vi "database MS Access test.vi"() -> ()   [LabVIEW 2020]
uses:
  source/Database OOP/Database Interfaces/Column Information.ctl
  source/Database OOP/Database Interfaces/Database data type.ctl
  source/Database OOP/ADODB/ADODB Class/ADODB.lvclass
  source/Database OOP/ADODB/UDL Connection Class/UDL Connection.lvclass
  C:/Users/User/Desktop/Raman Program/Database OOP/source/Database OOP/Database Interfaces/Database Connection Class/Database Connection.lvclass
  source/Database OOP/Database Interfaces/Database Advanced Schema Class/Database Adv Schema.lvclass
  source/Database OOP/Database Interfaces.lvlib
panel:
  out "Provider Name":string
  out "Timestamp":string[](array[string])
  out "Column Information Array 2":T1[](array[typedef])
  out "Primary Key Array":string[](array[string])
  out "Column Information Array":T1[](array[typedef])
  out "Foreign Key Array":T3(array[cluster])
  out "Column Name Array":string[](array[string])
  out "Table Names":string[](array[string])
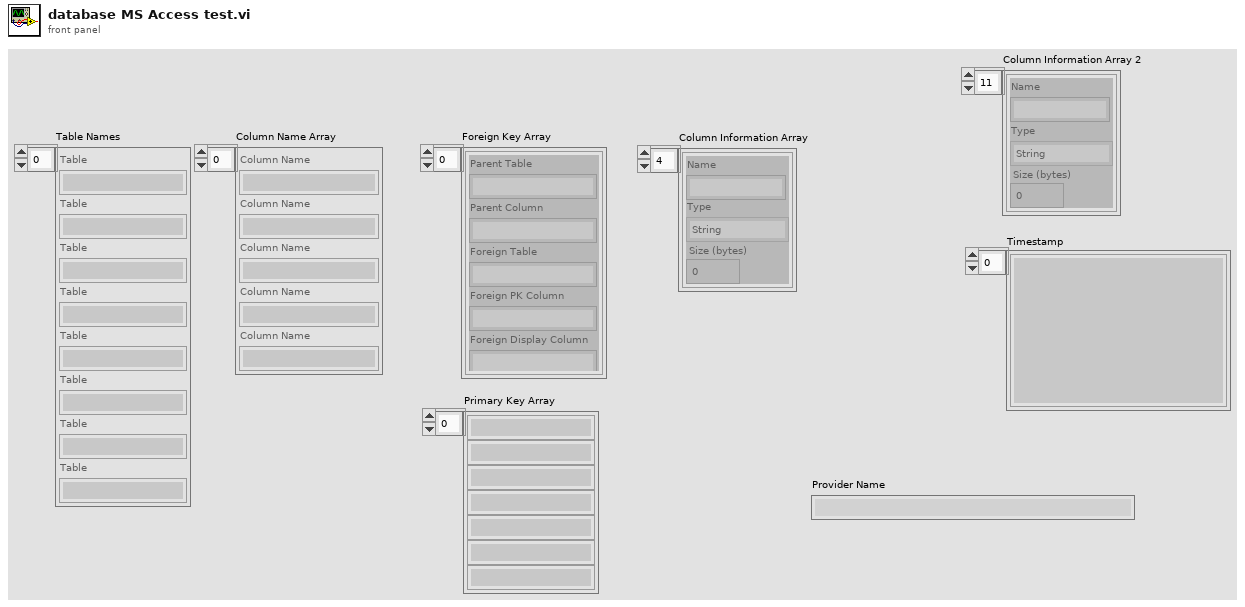
[diagram p1: front panel]
types:
  T1 = typedef "Database Interfaces.lvlib/Column Information.ctl" = cluster{"Name":string, "Type":T2, "Size (bytes)":i32}
  T2 = typedef "Database Interfaces.lvlib/Database data type.ctl" = enum16{"String", "Long (I32)", "Single (SGL)", "Double (DBL)", "Date/Time", "Binary"}
  T3 = cluster{"Parent Table":string, "Parent Column":string, "Foreign Table":string, "Foreign PK Column":string, "Foreign Display Column":string}[]
  T4 = typedef "Database Interfaces.lvlib/foreign key properties.ctl" = cluster{"FK Table":string, "FK Column":string, "PK Table":string, "PK Column":string, "PK Display Column":string}
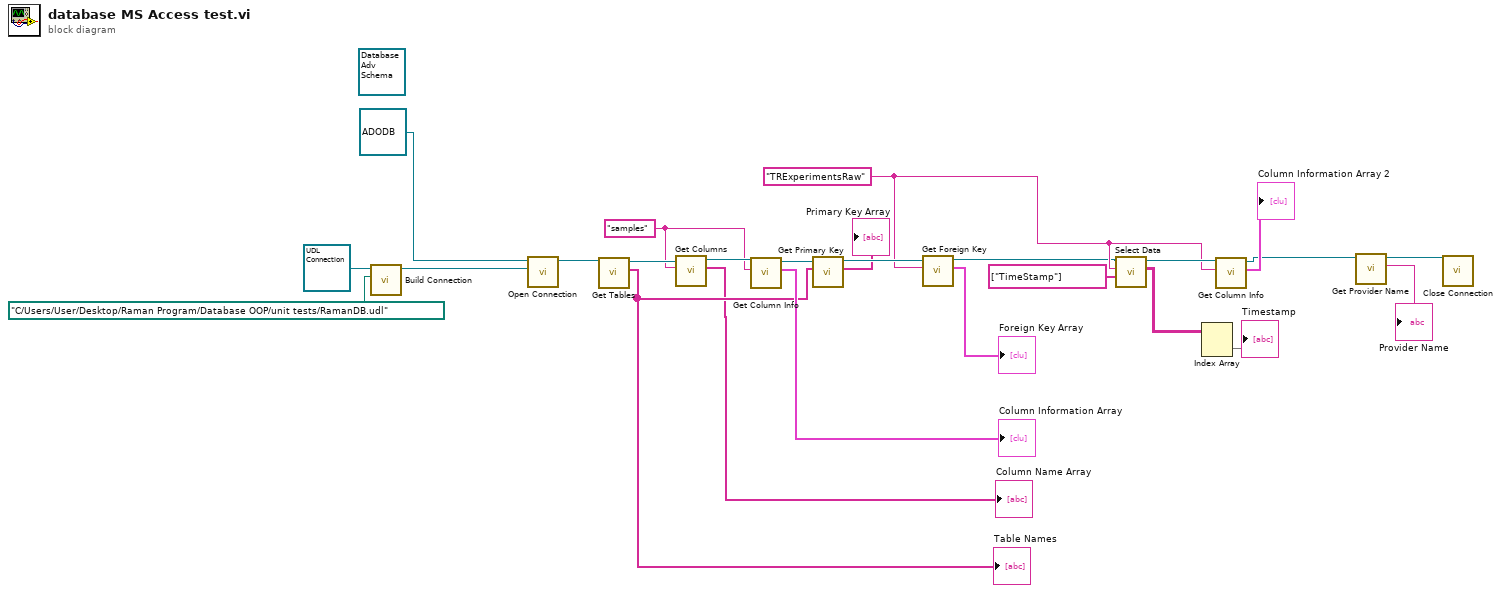
[diagram p0: block diagram]
diagram:
  (unwired) refnum<class "Database Adv Schema.lvclass"> refnum ("Database Interfaces.lvlib:Database Schema.lvclass")
  w9 = "TRExperimentsRaw" ("Table Name")
  w22 = "samples" ("Table Name")
  n1 = call "Build Connection.vi"("*.udl file path"=path "C:/Users/User/Desktop/Raman Program/Database OOP/unit tests/RamanDB.udl", "UDL Connection in"=refnum<class "UDL Connection.lvclass"> refnum ("ADODB.lvlib:UDL Connection.lvclass")) -> ("UDL Connection out"=w18:refnum<class "UDL Connection.lvclass">)  [unwired: 8 in, 1 out]
  n2 = call-dynamic "Open Connection.vi"("Connection"=w18, "ADODB in"=refnum<class "ADODB.lvclass"> refnum ("ODBC in")) -> ("ADODB out"=w25:refnum<class "ADODB.lvclass">)  [unwired: 8 in, 1 out]
  n3 = call-dynamic "Get Tables.vi"("ODBC in"=w25) -> ("Table Names"=w13:string[], "ODBC out"=w24:refnum<class "ADODB.lvclass">)  [unwired: 8 in, 1 out]
  "Table Names" <- w13
  n4 = call-dynamic "Get Columns.vi"("Table Name"=w22, "ADODB in"=w24) -> ("Column Name Array"=→"Column Name Array":string[], "ADODB out"=w23:refnum<class "ADODB.lvclass">)  [unwired: 7 in, 1 out]
  n5 = call-dynamic "Get Column Info.vi"("Table Name"=w22, "ODBC in"=w23) -> ("Column Information Array"=→"Column Information Array":T1[], "ODBC out"=w15:refnum<class "ADODB.lvclass">)  [unwired: 7 in, 1 out]
  n6 = call-dynamic "Get Primary Key.vi"("Table Name Array"=w13, "ADODB in"=w15) -> ("Primary Key Array"=→"Primary Key Array":string[], "ADODB out"=w14:refnum<class "ADODB.lvclass">)  [unwired: 6 in, 2 out]
  n7 = call-dynamic "Get Foreign Key.vi"("Table Name"=w9, "ADODB in"=w14) -> ("FK Properties Array"=→"Foreign Key Array":T4[], "ADODB out"=w7:refnum<class "ADODB.lvclass">)  [unwired: 7 in, 1 out]
  n8 = call-dynamic "Select Data.vi"("Columns"=string[] ["TimeStamp"], "Table"=w9, "ADODB in"=w7) -> ("Data"=w5:string[][], "ADODB out"=w10:refnum<class "ADODB.lvclass">)  [unwired: 6 in, 1 out]
  n9 = Index Array(array=w5) -> (element=→"Timestamp":string[])  [unwired: 2 in]
  n10 = call-dynamic "Get Column Info.vi"("Table Name"=w9, "ODBC in"=w10) -> ("Column Information Array"=→"Column Information Array 2":T1[], "ODBC out"=w3:refnum<class "ADODB.lvclass">)  [unwired: 7 in, 1 out]
  n11 = call-dynamic "Get Provider Name.vi"("ADODB in"=w3) -> ("Provider Name"=→"Provider Name":string, "ADODB out"=w2:refnum<class "ADODB.lvclass">)  [unwired: 8 in, 1 out]
  n12 = call-dynamic "Close Connection.vi"("ODBC in"=w2) -> ()  [unwired: 9 in, 2 out]
